vi "范围变换.vi"(0 "输入变换上限(2.2)":dbl=2.2, 1 "标度上限(2.02)":dbl=2.02, 2 "输入":dbl, 3 "输入变换下限(1.5)":dbl=1.5, 4 "标度下限(1.98)":dbl=1.98) -> (5 "输出":dbl)   [LabVIEW 2018]
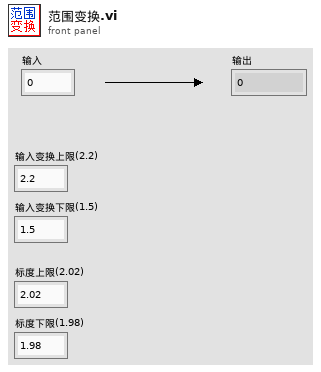
[diagram p1: front panel]
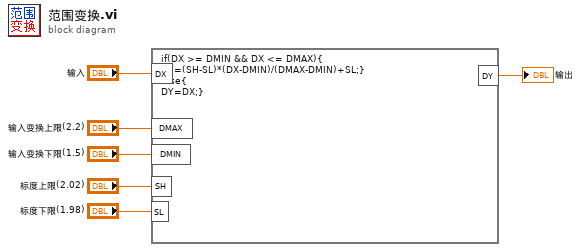
[diagram p0: block diagram]
diagram:
  n1 = formula code="if(DX >= DMIN && DX <= DMAX){\nDY=(SH-SL)*(DX-DMIN)/(DMAX-DMIN)+SL;}\nelse{\nDY=DX;}"("DX"="输入", "DMAX"="输入变换上限(2.2)", "DMIN"="输入变换下限(1.5)", "SH"="标度上限(2.02)", "SL"="标度下限(1.98)") -> ("DY"=→"输出":dbl)
